vi "Solenoid stuff.vi"() -> ()   [LabVIEW 2017]
uses:
  <vilib>/Rock Robotics/WPI/Solenoid/WPI_SolenoidValue.ctl
  <vilib>/Rock Robotics/WPI/Utilities/WPI_GetSetVariantRefNum.vi
  <vilib>/Rock Robotics/WPI/Solenoid/WPI_SolenoidSetEnum.vi
panel:
  out "Compressor Running":bool
  out "Compressor Enabled":bool
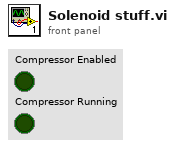
[diagram p1: front panel]
types:
  T1 = typedef "WPI_SolenoidValue.ctl" = enum16{"Off", "On", "Forward", "Reverse"}
  T2 = typedef "WPI_CompressorDevRef.ctl" = cluster{"DevStatus":errorcluster, "Pneumatics Control Module":u8}
  T3 = typedef "WPI_JoystickDevRef.ctl" = cluster{"Device":T4}
  T4 = typedef "WPI_JoystickDeviceEnum.ctl" = enum16{"USB 0", "USB 1", "USB 2", "USB 3", "USB 4", "USB 5"}
  T5 = typedef "WPI_SolenoidDevRef.ctl" = cluster{"DevStatus":errorcluster, "Pneumatics Control Module":u8, "Forward Solenoid Channel":T6, "Reverse Solenoid Channel":T6}
  T6 = typedef "WPI_SolenoidChannel.ctl" = enum8{"Solenoid 0", "Solenoid 1", "Solenoid 2", "Solenoid 3", "Solenoid 4", "Solenoid 5", "Solenoid 6", "Solenoid 7", "Invalid"}
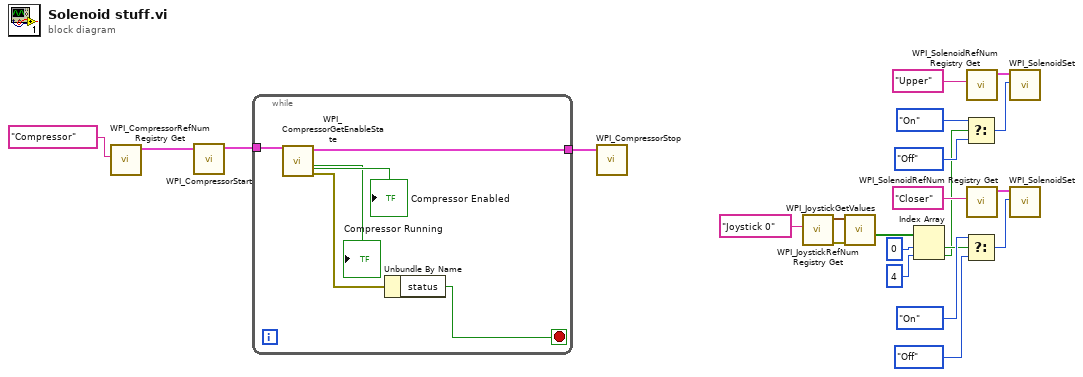
[diagram p0: block diagram]
diagram:
  n1 = call <vilib>:"WPI_CompressorRefNum Registry Get.vi"("refnum name"="Compressor") -> ("CompressorDevRef"=w4:T2)  [unwired: 9 in, 1 out]
  n2 = call <vilib>:"WPI_CompressorStart.vi"("CompressorDevRef"=w4) -> ("CompressorDevRef"=w2:T2)  [unwired: 9 in, 1 out]
  n3 = while {
    tunnel: w2 -> [w24]
    tunnel: [w23] -> w1
    stop <- w25 stop-if-true
    n4 = call <vilib>:"WPI_CompressorGetEnableState.vi"("CompressorDevRef"=w24) -> ("error out"=w26:errorcluster, "Compressor Running"=→"Compressor Running":bool, "Enabled"=→"Compressor Enabled":bool, "CompressorDevRef"=w23:T2)  [unwired: 7 in]
    n5 = Unbundle By Name(w26) -> ("status"=w25:bool)
  }
  n6 = call <vilib>:"WPI_CompressorStop.vi"("CompressorDevRef"=w1) -> ()  [unwired: 9 in, 2 out]
  n7 = call <vilib>:"WPI_JoystickRefNum Registry Get.vi"("refnum name"="Joystick 0") -> ("error out"=w16:errorcluster, "JoystickDevRef"=w17:T3)  [unwired: 9 in]
  n8 = call <vilib>:"WPI_JoystickGetValues.vi"("error in (no error)"=w16, "JoystickDevRef"=w17) -> ("Buttons"=w15:bool[])  [unwired: 5 in, 4 out]
  n9 = Index Array(array=w15, index #1=0 ("index"), index #2=4 ("index")) -> (element #1=w8:bool, element #2=w7:bool)
  n10 = Select(t=WPI_SolenoidValue."On" ("Value"), s=w7, f=WPI_SolenoidValue."Off" ("Value")) -> (s? t:f=w5:T1)
  n11 = Select(t=WPI_SolenoidValue."On" ("Value"), s=w8, f=WPI_SolenoidValue."Off" ("Value")) -> (s? t:f=w6:T1)
  n12 = call <vilib>:"WPI_SolenoidRefNum Registry Get.vi"("refnum name"="Upper") -> ("SolenoidDevRef"=w19:T5)  [unwired: 9 in, 1 out]
  n13 = call <vilib>:"WPI_SolenoidRefNum Registry Get.vi"("refnum name"="Closer") -> ("SolenoidDevRef"=w20:T5)  [unwired: 9 in, 1 out]
  n14 = call-poly <vilib>:"WPI_SolenoidSet.vi"("Value"=w5, "SolenoidDevRef"=w19) -> ()  [unwired: 8 in, 2 out]
  n15 = call-poly <vilib>:"WPI_SolenoidSet.vi"("Value"=w6, "SolenoidDevRef"=w20) -> ()  [unwired: 8 in, 2 out]
